vi "Report Type.vi"(0 "report in":refnum<class "NI_report.lvclass">, 11 "error in (no error)":errorcluster) -> (4 "report out":refnum<class "NI_report.lvclass">, 8 "report type":T1, 15 "error out":errorcluster)   [LabVIEW 2020, in "NI_report.lvclass"]
doc: "Returns the report type, such as HTML, of a specified report."
uses:
  NI_report.lvclass
  Report Type.ctl
  NI_ReportGenerationCore.lvlib
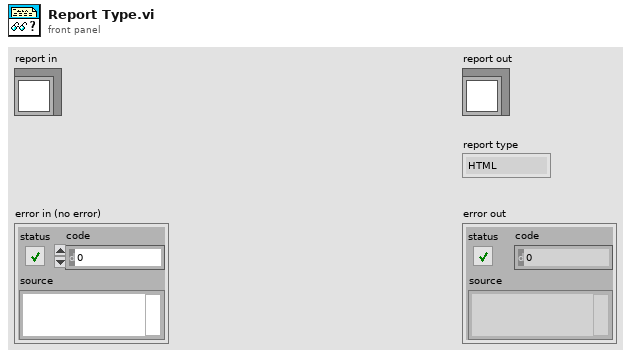
[diagram p1: front panel]
types:
  T1 = typedef "NI_ReportGenerationCore.lvlib/Report Type.ctl" = enum16{"HTML", "Word", "Excel"}
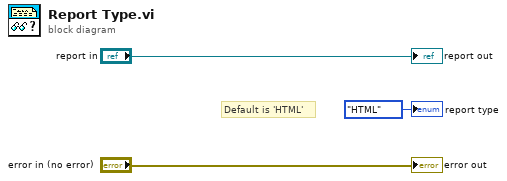
[diagram p0: block diagram]
diagram:
  # "Default is 'HTML'"
  "error out" <- "error in (no error)"
  "report out" <- "report in"
  "report type" <- Report_Type."HTML" ("report type")
